vi "measure_2614_lxy.vi"(11 "2614 resource name":refnum<visa-resource-name>) -> (2 "输出数组":string[](array[string]), 3 "2641 resource name out":refnum<visa-resource-name>)   [LabVIEW 2019]
uses:
  <vilib>/Analysis/baseanly.llb/Mean (DBL).vi
  lib/Keithley 2600 Series/Public/Data/Read Measurement (Resistance).vi
  <vilib>/Analysis/NI_AALBase.lvlib
  lib/Keithley 2600 Series/Keithley 2600 Series.lvlib
panel:
  out "error out 2":errorcluster caption="错误输出 2"
  in  "error out":errorcluster
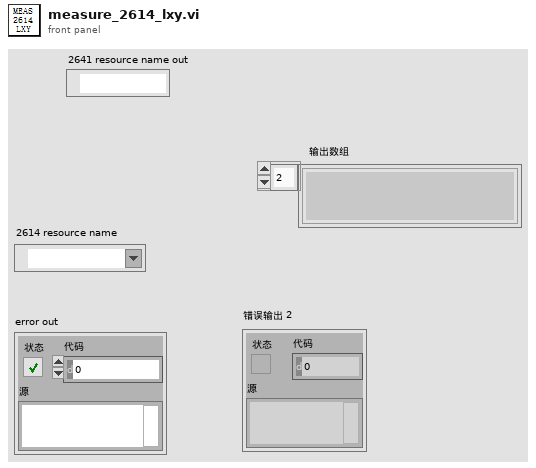
[diagram p1: front panel]
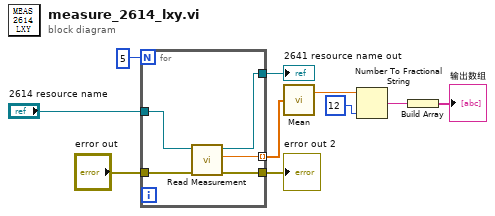
[diagram p0: block diagram]
diagram:
  n1 = for {
    N: 5 -> [_]
    tunnel: [w13] -> w9 mode=indexing
    tunnel: [w11] -> w3
    tunnel: "error out" -> [w14]
    tunnel: [w12] -> w2
    tunnel: "2614 resource name" -> [w15]
    n2 = call-poly "Read Measurement.vi"("error in (no error)"=w14, "VISA resource name"=w15) -> ("error out"=w11:errorcluster, "Last Resistance (Ohm)"=w13:dbl, "VISA resource name out"=w12:refnum<visa-resource-name>)  [unwired: 6 in, 1 out]
  }
  "error out 2" <- w3
  "2641 resource name out" <- w2
  n3 = call-poly <vilib>:"Mean.vi"("X"=w9) -> ("mean"=w8:dbl)  [unwired: 1 out]
  n4 = Number To Fractional String(number=w8, precision (6)=i16 12 ("精度(6)")) -> (F-format string=w6:string)  [unwired: 2 in]
  n5 = Build Array(w6) -> (→"输出数组":string[])
